vi "Call And Receive Multiple.vi"(6 "timeout in ms (-1)":i32=-1, 8 "error in (no error)":errorcluster, 9 "Parameter":variant[](array[variant]), 10 "Function":string[](array[string]), 11 "input in":refnum<class "Input.lvclass">) -> (0 "error out":errorcluster, 1 "timeout":bool[](array[boolean]), 2 "Data":variant[](array[variant]), 3 "input out":refnum<class "Input.lvclass">)   [LabVIEW 2015, in "Input.lvclass"]
uses:
  Input.lvclass
  Result/result_from_call/result_from_call.lvclass
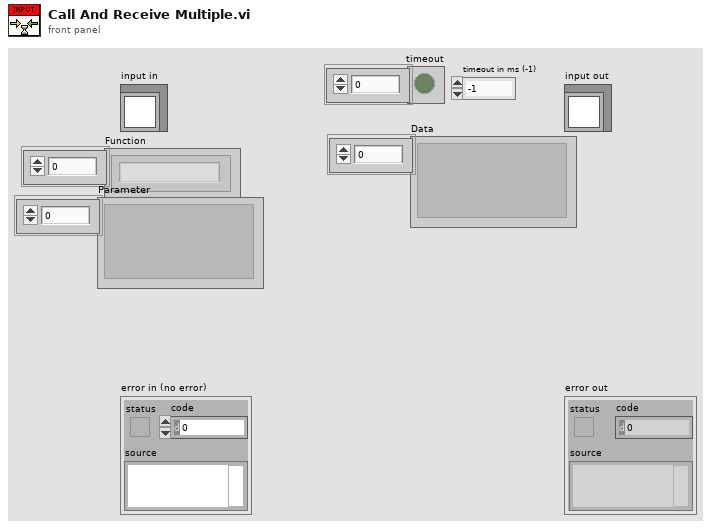
[diagram p1: front panel]
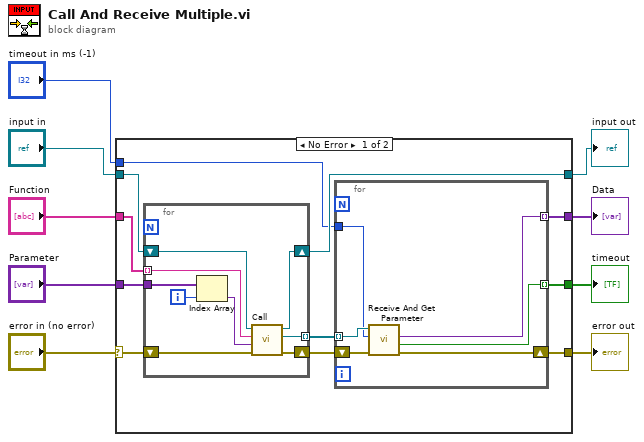
[diagram p0: block diagram]
diagram:
  n1 = case shown="No Error" "error in (no error)" {
    selector: "error in (no error)" -> [w10 w37]
    tunnel: [w15 w37] -> w8
    tunnel: [w12 w36] -> w6
    tunnel: "input in" -> [w16 w36]
    tunnel: "Parameter" -> [w17 _]
    tunnel: "Function" -> [w18 _]
    tunnel: [w14 _] -> w3
    tunnel: [w13 _] -> w2
    tunnel: "timeout in ms (-1)" -> [w11 _]
    frame No Error {
      n2 = for {
        tunnel: [w35] -> w20 mode=indexing
        tunnel: w18 -> [w33] mode=indexing
        tunnel: w17 -> [w29]
        shift-right: [w31] -> w12
        shift-left: w16 -> [w32]
        shift-right: [w34] -> w19
        shift-left: w10 -> [w30]
        i -> [w27]
        n3 = Index Array(array=w29, index=w27) -> (element=w28:variant)
        n4 = call "Call.vi"("error in (no error)"=w30, "Parameter"=w28, "Function"=w33, "input in"=w32) -> ("error out"=w34:errorcluster, "result"=w35:refnum<class "result_from_call.lvclass">, "input out"=w31:refnum<class "Input.lvclass">)  [unwired: 5 in]
      }
      n5 = for {
        tunnel: w20 -> [w26] mode=indexing
        tunnel: [w23] -> w14 mode=indexing
        tunnel: [w22] -> w13 mode=indexing
        tunnel: w11 -> [w21]
        shift-right: [w24] -> w15
        shift-left: w19 -> [w25]
        n6 = call "Receive And Get Parameter.vi"("error in (no error)"=w25, "timeout in ms (-1)"=w21, "result_from_call in"=w26) -> ("error out"=w24:errorcluster, "timeout"=w23:bool, "Data"=w22:variant)  [unwired: 5 in, 1 out]
      }
    }
    frame Error {
    }
  }
  "error out" <- w8
  "input out" <- w6
  "Data" <- w2
  "timeout" <- w3
